vi "Persistence value.vi"(1 "Persistence In":bool, 2 "Read/Write this vi":bool) -> (0 "Persistence Out":bool)   [LabVIEW 2019]
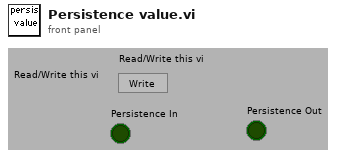
[diagram p1: front panel]
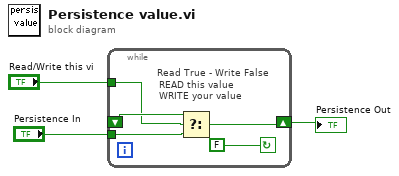
[diagram p0: block diagram]
diagram:
  n1 = while {
    shift-right: [w7] -> w1
    shift-left: _ -> [w8]
    tunnel: "Read/Write this vi" -> [w4]
    tunnel: "Persistence In" -> [w6]
    stop <- FALSE continue-if-true
    # "READ this value\nWRITE your value"
    # "Read True - Write False"
    n2 = Select(t=w8, s=w4, f=w6) -> (s? t:f=w7:bool)
  }
  "Persistence Out" <- w1
